vi "난수발생(VI 서버).vi"(4 "가운데로":bool, 6 "메뉴바/도구바":bool, 7 "정지":bool, 11 "난수 발생":bool) -> (2 "웨이브폼 차트":dbl(graph))   [LabVIEW 2014]
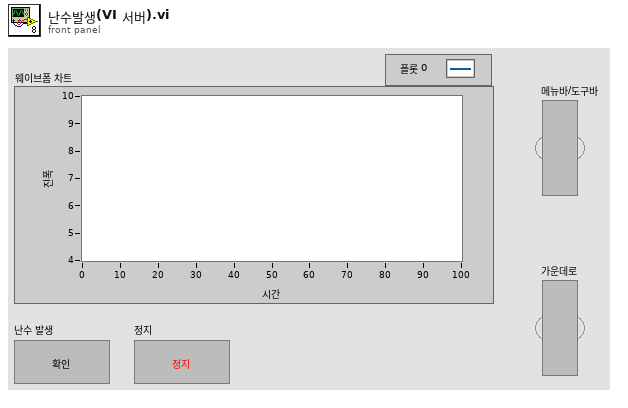
[diagram p1: front panel]
types:
  T1 = enum16{"Always On", "Always Off", "Off While Running"}
  T2 = enum32{"invalid app kind", "Development System", "Run Time System", "Student Edition", "Embedded LabVIEW", "Evaluation", "Custom"}
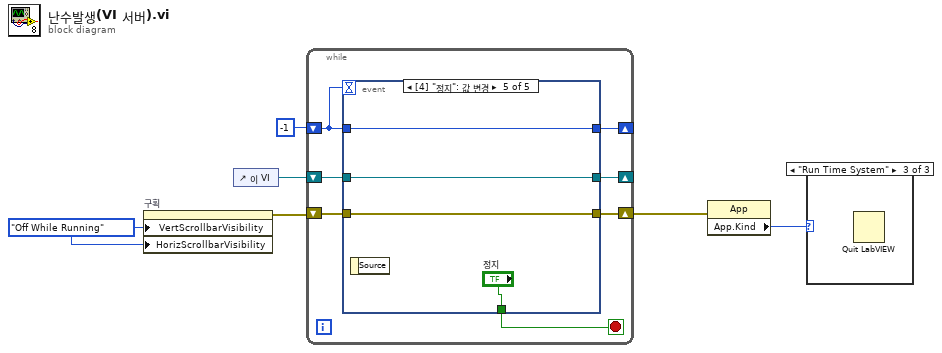
[diagram p0: block diagram]
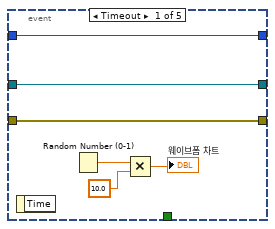
[diagram p4: hidden frame]
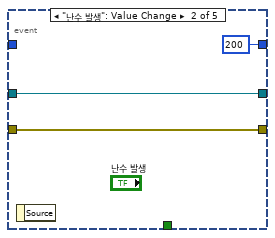
[diagram p5: hidden frame]
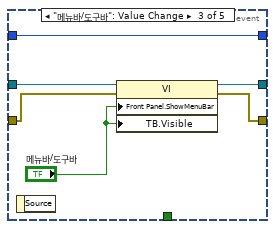
[diagram p6: hidden frame]
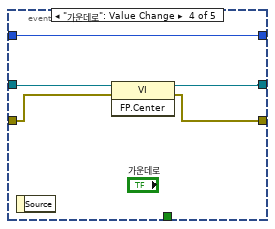
[diagram p7: hidden frame]
diagram:
  w4 = T1."Off While Running" ("수직 스크롤 막대 보이기")
  n1 = property on="구획" class="Pane"("VertScrollbarVisibility"=w4, "HorizScrollbarVisibility"=w4) -> (error out=w3:errorcluster)  [unwired: 2 in, 1 out]
  n2 = control-ref of="이 VI"() -> (w5:refnum<vi>)
  n3 = while {
    shift-right: [w12] -> _
    shift-left: -1 -> [w13]
    shift-right: [w8] -> _
    shift-left: w5 -> [w10]
    shift-right: [w7] -> w2
    shift-left: w3 -> [w9]
    stop <- w11 stop-if-true
    n4 = event shown="[4] \"정지\": 값 변경" {
      selector: _ -> [_ _ _ _ _]
      dyn-events: _ -> [_ _ _ _ _]
      timeout: w13 -> [_ _ _ _ _]
      tunnel: [w19 200 w28 w33 w36] -> w12
      tunnel: w13 -> [w19 _ w28 w33 w36]
      tunnel: [_ _ _ _ "정지"] -> w11
      tunnel: w10 -> [w15 w22 w26 w32 w35]
      tunnel: w9 -> [w14 w21 w25 w30 w34]
      tunnel: [w15 w22 w27 w31 w35] -> w8
      tunnel: [w14 w21 w24 w29 w34] -> w7
      event Timeout {
        n5 = event-data() -> ()  [unwired: 1 in, 1 out]
        n6 = Random Number (0-1)() -> (number: 0 to 1=w17:dbl)
        n7 = Multiply(x=w17, y=10.0) -> (x*y=→"웨이브폼 차트":dbl)
      }
      event "난수 발생": Value Change {
        n8 = event-data() -> ()  [unwired: 1 in, 1 out]
      }
      event "메뉴바/도구바": Value Change {
        n9 = event-data() -> ()  [unwired: 1 in, 1 out]
        n10 = property class="VI"(reference=w26, error in=w25, "Front Panel.ShowMenuBar"="메뉴바/도구바", "TB.Visible"="메뉴바/도구바") -> (reference out=w27:refnum<vi>, error out=w24:errorcluster)
      }
      event "가운데로": Value Change {
        n11 = event-data() -> ()  [unwired: 1 in, 1 out]
        n12 = invoke class="VI" method="FP.Center"(reference=w32, error in=w30) -> (reference out=w31:refnum<vi>, error out=w29:errorcluster)  [unwired: 1 in, 1 out]
      }
      event "정지": Value Change {
        n13 = event-data() -> ()  [unwired: 1 in, 1 out]
      }
    }
  }
  n14 = property class="App"(error in=w2) -> ("App.Kind"=w1:T2)  [unwired: 1 in, 2 out]
  n15 = case shown="\"Run Time System\"" w1 {
    frame "invalid app kind", Default {
    }
    frame "Development System" {
    }
    frame "Run Time System" {
      n16 = Quit LabVIEW() -> ()  [unwired: 1 in]
    }
  }
